vi "generate_DAC_voltages_V1_withPockels.vi"(7 "focus mode?":bool, 8 "derived values":T1, 9 "scan specification":T4={"x amplitude"=0, "x resolution (pixels)"=0, "x offset fly-forward (iterations)"=0, "x offset fly-back (iterations)"=0, "y resolution (nr. of lines)"=0, "y step size"=0, "iterations per pixel"=0, "number of frames"=0, "y offset (pixels)"=0, "number of y-brake lines  (before y-fly-back)"=0, "number y-brake lines (after y-fly-back)"=0, "number of y-fly-back steps"=8, "lines per z step"=0, "number of z/intensity tuples"=0, "number of repetitions (volumes or planes)"=0, "z step size derived"=0, "choose the beginning of z scan"=FALSE, "number of frames (settings)"=0, "FPGA trajectory?"=FALSE, "Pockels cell voltage (bits)"=0}, 10 "counter cluster in":T2, 11 "resonant trigger":bool) -> (0 "acquire?":bool, 1 "fly-back acquisition phase?":bool, 2 "counter cluster out":T2, 3 "DAC voltages":T3 {"ch6" max=4095 step=1; "ch5" max=4095 step=1; "ch4" max=4095 step=1; "ch3" max=4095 step=1; "ch2" max=4095 step=1; "ch1" max=4095 step=1; "ch0" max=4095 step=1})   [LabVIEW 2010]
uses:
  scan_specification_cluster.ctl
  common_typedefs/DAC_voltage_cluster.ctl
  counter_cluster.ctl
  derived_values_cluster.ctl
panel:
  out "coerced(x)":u16
  out "coerced(x) 2":u16
  out "unsigned 16bit integer":u16
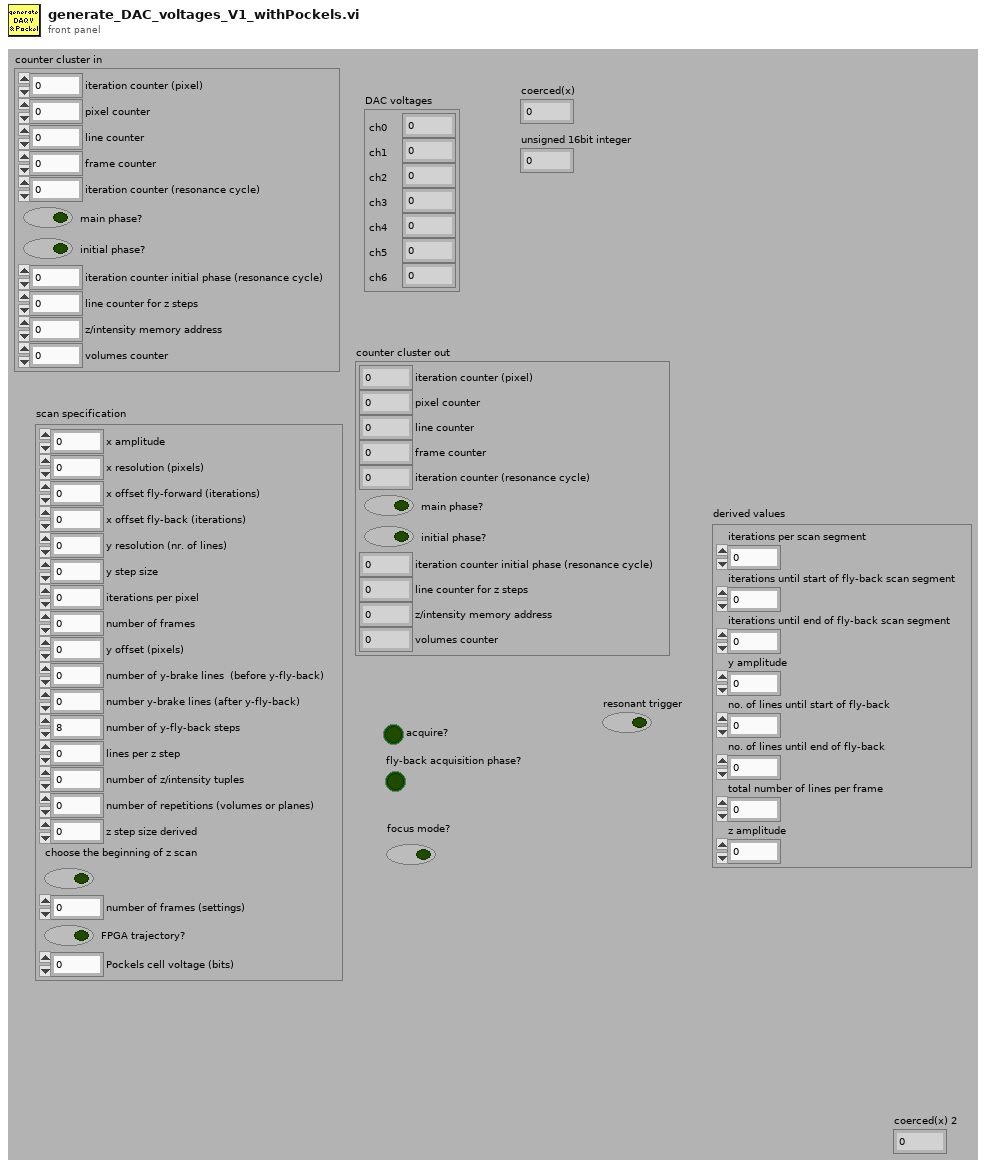
[diagram p1: front panel]
types:
  T1 = typedef "derived_values_cluster.ctl" = cluster{"iterations per scan segment":u16, "iterations until start of fly-back scan segment":u16, "iterations until end of fly-back scan segment":u16, "y amplitude":u16, "no. of lines until start of fly-back":u16, "no. of lines until end of fly-back":u16, "total number of lines per frame ":u16, "z amplitude":u16}
  T2 = typedef "counter_cluster.ctl" = cluster{"iteration counter (pixel)":u16, "pixel counter":u16, "line counter":u16, "frame counter":u16, "iteration counter (resonance cycle)":u16, "main phase?":bool, "initial phase?":bool, "iteration counter initial phase (resonance cycle)":u16, "line counter for z steps":u16, "z/intensity memory address":u32, "volumes counter":u16}
  T3 = typedef "DAC_voltage_cluster.ctl" = cluster{"ch0":u16, "ch1":i16, "ch2":i16, "ch3":i16, "ch4":u16, "ch5":u16, "ch6":u16}
  T4 = typedef "scan_specification_cluster.ctl" = cluster{"x amplitude":u16, "x resolution (pixels)":u16, "x offset fly-forward (iterations)":u16, "x offset fly-back (iterations)":u16, "y resolution (nr. of lines)":u16, "y step size":u16, "iterations per pixel":u16, "number of frames":i32, "y offset (pixels)":u16, "number of y-brake lines  (before y-fly-back)":u16, "number y-brake lines (after y-fly-back)":u16, "number of y-fly-back steps":u16, "lines per z step":u16, "number of z/intensity tuples":u16, "number of repetitions (volumes or planes)":i32, "z step size derived":u16, "choose the beginning of z scan":bool, "number of frames (settings)":i32, "FPGA trajectory?":bool, "Pockels cell voltage (bits)":i16}
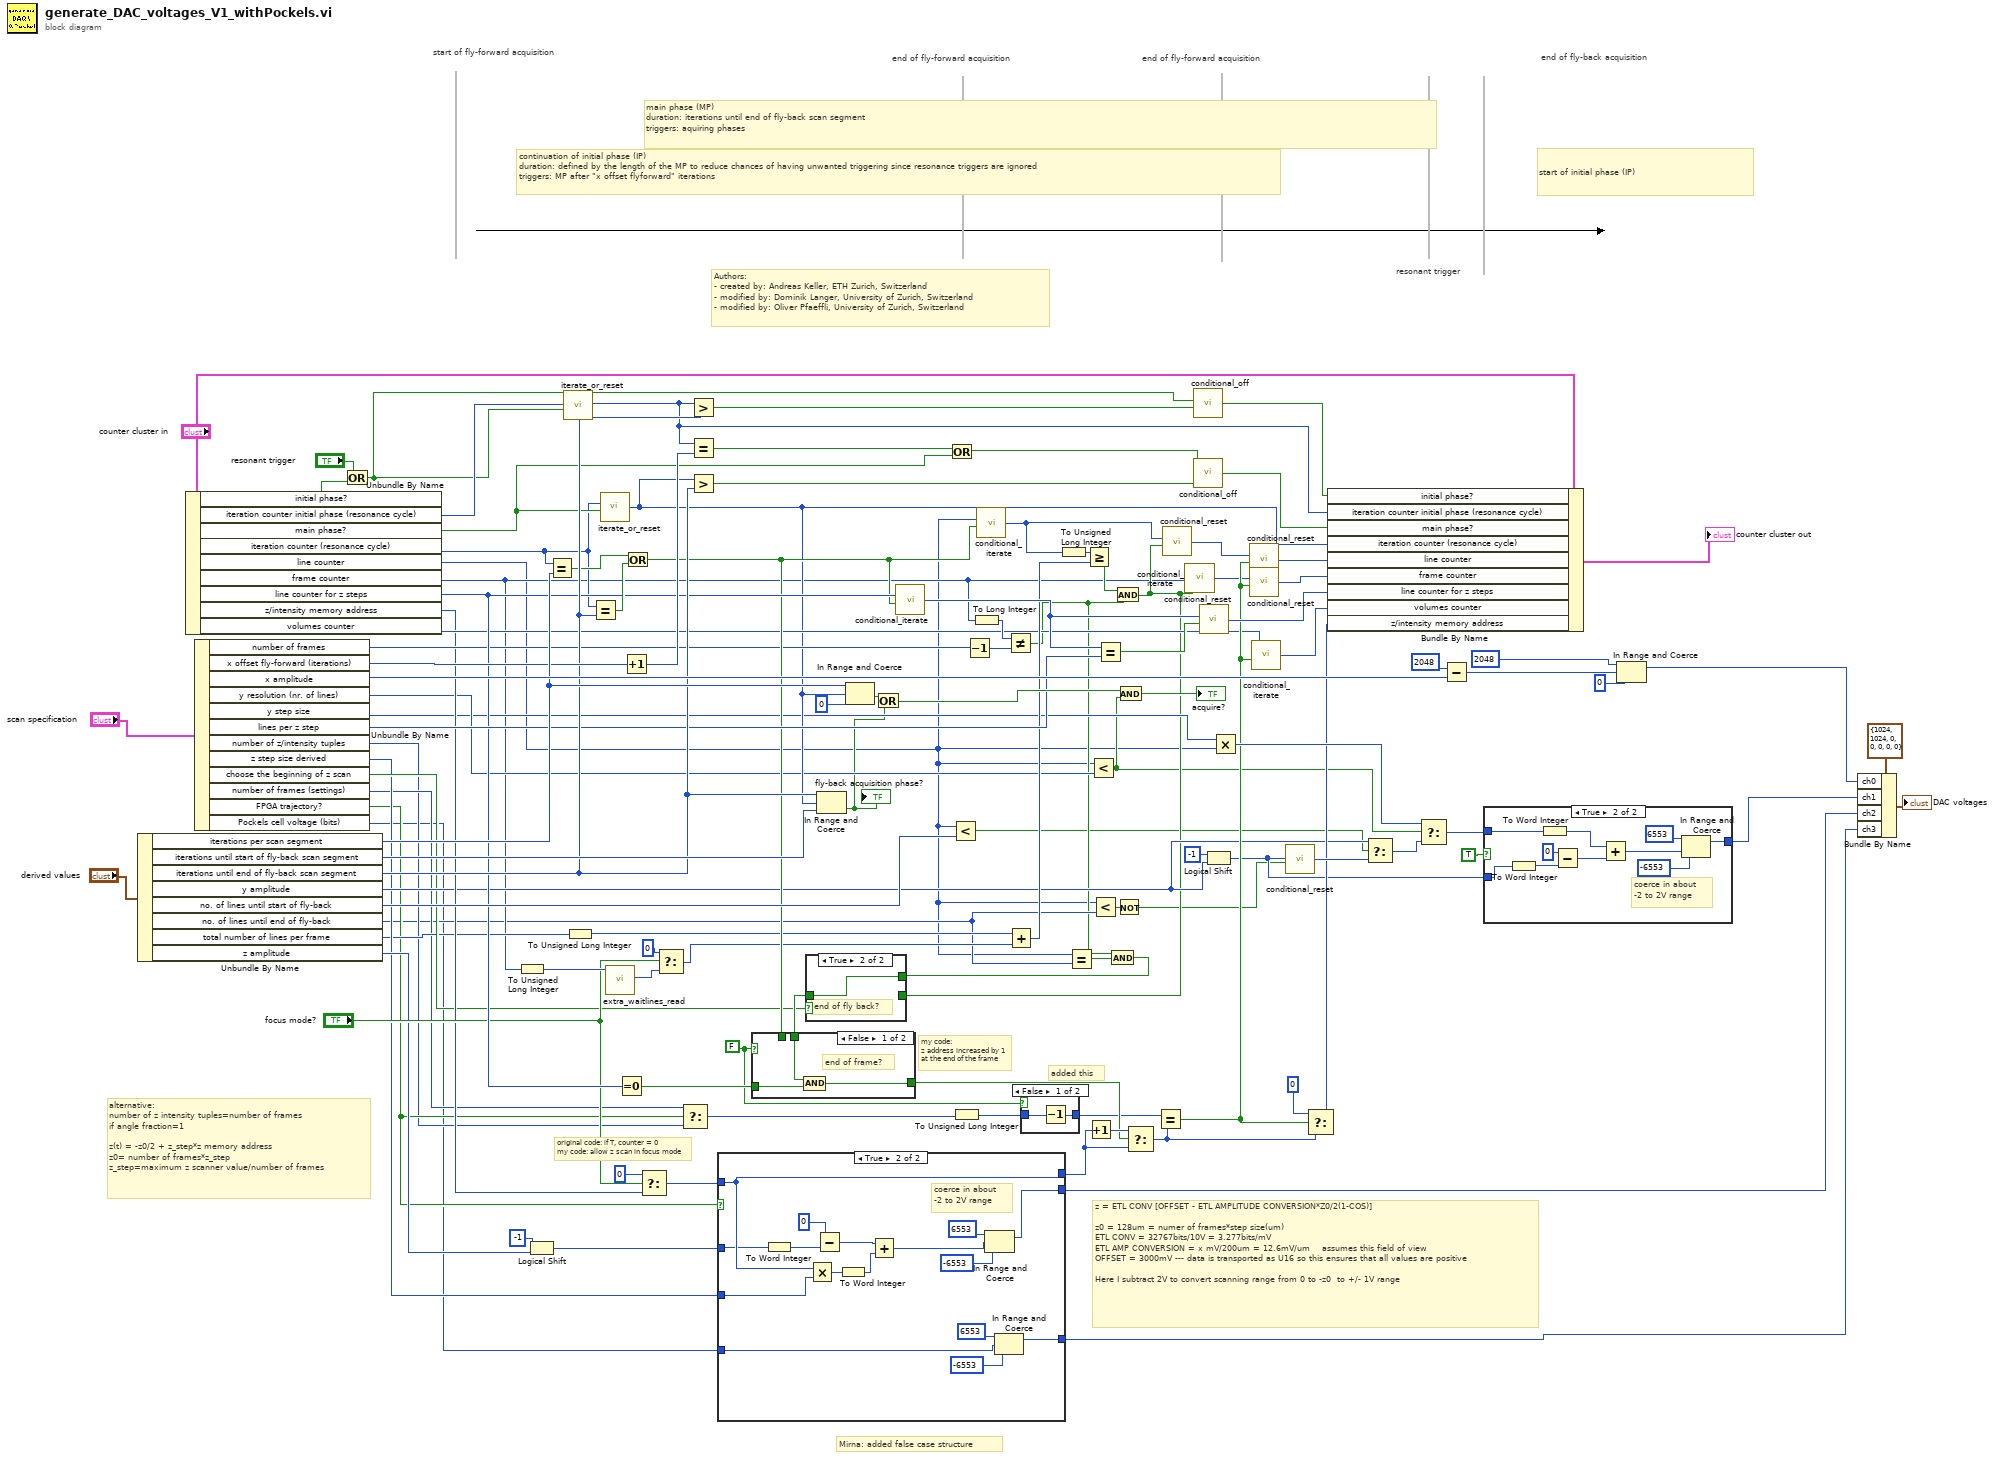
[diagram p0: block diagram]
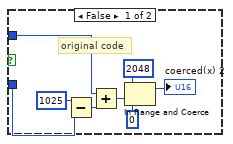
[diagram p3: hidden frame]
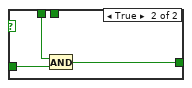
[diagram p5: hidden frame]
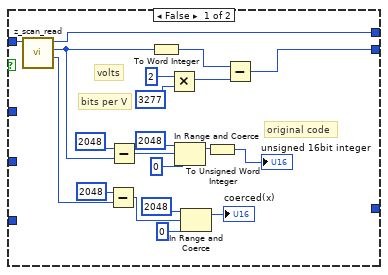
[diagram p6: hidden frame]
diagram:
  w6 = FALSE
  # "added this"
  # "z = ETL CONV [OFFSET - ETL AMPLITUDE CONVERSION*Z0/2(1-COS)]\n\nz0 = 128um = numer of frames*step size(um)\nETL CONV = 32767bits/10V = 3.277bits/mV\nETL AMP CONVERSION = x mV/200um = 12.6mV/um    assumes this field of view\nOFFSET = 3000mV --- data is transported as U16 so this ensures that all values are positive\n\nHere I subtract 2V to convert scanning range from 0 to -z0  to +/- 1V range"
  # "my code:\nz address increased by 1\nat the end of the frame"
  # "alternative:\nnumber of z intensity tuples=number of frames\nif angle fraction=1\n\nz(t) = -z0/2 + z_step*z memory address\nz0= number of frames*z_step\nz_step=maximum z scanner value/number of frames"
  # "original code: if T, counter = 0\nmy code: allow z scan in focus mode"
  # "Mirna: added false case structure"
  # "start of initial phase (IP)"
  # "continuation of initial phase (IP)\nduration: defined by the length of the MP to reduce chances of having unwanted triggering since resonance triggers are ignored\ntriggers: MP after \"x offset flyforward\" iterations"
  # "end of fly-back acquisition"
  # "end of fly-forward acquisition"
  # "end of fly-forward acquisition"
  # "start of fly-forward acquisition"
  # "main phase (MP)\nduration: iterations until end of fly-back scan segment\ntriggers: aquiring phases"
  # "resonant trigger"
  # "Authors: \n- created by: Andreas Keller, ETH Zurich, Switzerland\n- modified by: Dominik Langer, University of Zurich, Switzerland\n- modified by: Oliver Pfaeffli, University of Zurich, Switzerland"
  n1 = Unbundle By Name("derived values") -> ("iterations per scan segment"=w93:u16, "iterations until start of fly-back scan segment"=w96:u16, "iterations until end of fly-back scan segment"=w80:u16, "y amplitude"=w36:u16, "no. of lines until start of fly-back"=w84:u16, "no. of lines until end of fly-back"=w11:u16, "total number of lines per frame"=w29:u16, "z amplitude"=w34:u16)
  n2 = Unbundle By Name("counter cluster in") -> ("initial phase?"=w95:bool, "iteration counter initial phase (resonance cycle)"=w91:u16, "main phase?"=w47:bool, "iteration counter (resonance cycle)"=w39:u16, "line counter"=w5:u16, "frame counter"=w28:u16, "line counter for z steps"=w73:u16, "z/intensity memory address"=w42:u32, "volumes counter"=w52:u16)
  n3 = Unbundle By Name("scan specification") -> ("number of frames"=w59:i32, "x offset fly-forward (iterations)"=w83:u16, "x amplitude"=w100:u16, "y resolution (nr. of lines)"=w40:u16, "y step size"=w35:u16, "lines per z step"=w77:u16, "number of z/intensity tuples"=w13:u16, "z step size derived"=w30:u16, "choose the beginning of z scan"=w31:bool, "number of frames (settings)"=w14:i32, "FPGA trajectory?"=w15:bool, "Pockels cell voltage (bits)"=w1:i16)
  n4 = Or(x="resonant trigger", y=w95) -> (x .or. y?=w89:bool)
  n5 = To Unsigned Long Integer(number=w28) -> (unsigned 32bit integer=w65:u32)
  n6 = Logical Shift(y=i16 -1 ("n"), x=w34) -> (x << y=w49:u16)
  n7 = Equal?(x=w39, y=w93) -> (x = y?=w78:bool)
  n8 = call "iterate_or_reset.vi"("iterate?"=w89, "number in"=w91) -> ("number out"=w25:u16)  [unwired: 4 in]
  n9 = To Unsigned Long Integer(number=w29) -> (unsigned 32bit integer=w26:u32)
  n10 = Equal?(x=w39, y=w80) -> (x = y?=w79:bool)
  n11 = call "iterate_or_reset.vi"("iterate?"=w47, "number in"=w39) -> ("number out"=w46:u16)  [unwired: 4 in]
  n12 = call "extra_waitlines_read.vi"("address extra waitlines IN"=w65) -> ("extra waitline data"=w8:u32)  [unwired: 9 in, 1 out]
  n13 = Equal To 0?(x=w73) -> (x = 0?=w68:bool)
  n14 = Increment(x=w83) -> (x+1=w82:u16)
  n15 = Or(x=w78, y=w79) -> (x .or. y?=w67:bool)
  n16 = Select(t=u32 0, s="focus mode?", f=w42) -> (s? t:f=w43:u32)
  n17 = Select(t=u32 0, s="focus mode?", f=w8) -> (s? t:f=w54:u32)
  n18 = Select(t=w14, s=w15, f=w13) -> (s? t:f=w41:i32)
  n19 = Greater?(x=w25, y=w80) -> (0:w81:bool)
  n20 = Equal?(x=w25, y=w82) -> (x = y?=w90:bool)
  n21 = Greater?(x=w46, y=w80) -> (0:w87:bool)
  n22 = case shown="True" w15 {
    tunnel: [w134 w148] -> w66
    tunnel: [w119 w139] -> w44
    tunnel: w43 -> [w133 w148]
    tunnel: w49 -> [_ w140]
    tunnel: w30 -> [_ w149]
    tunnel: [_ w136] -> w3
    tunnel: w1 -> [_ w135]
    frame False {
      # "bits per V"
      # "volts"
      # "original code"
      n23 = call "z_scan_read.vi"("address in"=w133) -> ("intensity"=w130:u16, "z-value"=w121:i16, "address out"=w134:u32)  [unwired: 8 in]
      n24 = Subtract(x=i16 2048, y=w130) -> (x-y=w127:u16)
      n25 = Subtract(x=i16 2048, y=w121) -> (x-y=w123:i16)
      n26 = To Word Integer(number=w121) -> (16bit integer=w120:i16)
      n27 = Multiply(x=i16 2 ("y"), y=i16 3277) -> (x*y=w117:i16)
      n28 = In Range and Coerce(upper limit=i16 2048, x=w123, lower limit=i16 0) -> (coerced(x)=w124:i16)  [unwired: 1 out]
      n29 = In Range and Coerce(upper limit=u16 2048, x=w127, lower limit=u16 0) -> (coerced(x)=→"coerced(x)":u16)  [unwired: 1 out]
      n30 = To Unsigned Word Integer(number=w124) -> (unsigned 16bit integer=→"unsigned 16bit integer":u16)
      n31 = Subtract(x=w120, y=w117) -> (x-y=w119:i16)
    }
    frame True {
      # "coerce in about\n-2 to 2V range"
      n32 = To Word Integer(number=w140) -> (16bit integer=w145:i16)
      n33 = Multiply(x=w148, y=w149) -> (x*y=w146:u32)
      n34 = Subtract(x=i16 0, y=w145) -> (x-y=w147:i16)
      n35 = To Word Integer(number=w146) -> (16bit integer=w144:i16)
      n36 = Add(x=w147, y=w144) -> (x+y=w141:i16)
      n37 = In Range and Coerce(upper limit=i16 6553, x=w141, lower limit=i16 -6553) -> (coerced(x)=w139:i16)  [unwired: 1 out]
      n38 = In Range and Coerce(upper limit=i16 6553, x=w135, lower limit=i16 -6553) -> (coerced(x)=w136:i16)  [unwired: 1 out]
    }
  }
  n39 = In Range and Coerce(upper limit=w80, x=w46, lower limit=w96) -> (In Range?=w18:bool)  [unwired: 1 out]
  "fly-back acquisition phase?" <- w18
  n40 = In Range and Coerce(upper limit=w93, x=w46, lower limit=u16 0) -> (In Range?=w108:bool)  [unwired: 1 out]
  n41 = Or(x=w108, y=w18) -> (x .or. y?=w99:bool)
  n42 = call "conditional_iterate.vi"("iterate?"=w67, "number in"=w73) -> ("number out"=w74:u16)  [unwired: 4 in]
  n43 = Or(x=w90, y=w47) -> (x .or. y?=w48:bool)
  n44 = Less?(x=w5, y=w84) -> (x < y?=w2:bool)
  n45 = To Unsigned Long Integer(number=w41) -> (unsigned 32bit integer=w71:u32)
  n46 = Decrement(x=w59) -> (x-1=w58:i32)
  n47 = To Long Integer(number=w28) -> (32bit integer=w57:i32)
  n48 = call "conditional_iterate.vi"("iterate?"=w67, "number in"=w5) -> ("number out"=w10:u16)  [unwired: 4 in]
  n49 = Not Equal?(x=w57, y=w58) -> (x != y?=w9:bool)
  n50 = Add(x=w26, y=w54) -> (x+y=w55:u32)
  n51 = case shown="False" w6 {
    tunnel: w71 -> [w152 w153]
    tunnel: [w151 w153] -> w7
    frame False {
      n52 = Decrement(x=w152) -> (x-1=w151:u32)
    }
    frame True {
    }
  }
  n53 = To Unsigned Long Integer(number=w10) -> (unsigned 32bit integer=w12:u32)
  n54 = Equal?(x=w5, y=w11) -> (x = y?=w16:bool)
  n55 = Greater Or Equal?(x=w12, y=w55) -> (x >= y?=w60:bool)
  n56 = Increment(x=w66) -> (x+1=w72:u32)
  n57 = Less?(x=w5, y=w40) -> (x < y?=w21:bool)
  n58 = Less?(x=w5, y=w11) -> (x < y?=w98:bool)
  n59 = Equal?(x=w74, y=w77) -> (x = y?=w75:bool)
  n60 = And(x=w9, y=w16) -> (x .and. y?=w17:bool)
  n61 = And(x=w60, y=w9) -> (x .and. y?=w33:bool)
  n62 = case shown="True" w31 {
    tunnel: w17 -> [_ w155]
    tunnel: w33 -> [w154 _]
    tunnel: [w154 w155] -> w32
    frame False {
      # "end of frame?"
    }
    frame True {
      # "end of fly back?"
    }
  }
  n63 = case shown="False" w6 {
    tunnel: w68 -> [w158 w161]
    tunnel: w67 -> [_ w160]
    tunnel: [w157 w159] -> w27
    tunnel: w32 -> [w156 _]
    frame False {
      # "end of frame?"
      n64 = And(x=w156, y=w158) -> (x .and. y?=w157:bool)
    }
    frame True {
      n65 = And(x=w160, y=w161) -> (x .and. y?=w159:bool)
    }
  }
  n66 = Not(x=w98) -> (.not. x?=w19:bool)
  n67 = And(x=w99, y=w21) -> (x .and. y?=→"acquire?":bool)
  n68 = Select(t=w72, s=w27, f=w66) -> (s? t:f=w70:u32)
  n69 = Equal?(x=w7, y=w70) -> (x = y?=w56:bool)
  n70 = call "conditional_reset.vi"("reset?"=w33, "number in"=w10) -> ("number out"=w62:u16)  [unwired: 4 in]
  n71 = call "conditional_iterate.vi"("iterate?"=w33, "number in"=w28) -> ("number out"=w37:u16)  [unwired: 4 in]
  n72 = call "conditional_off.vi"("switch off?"=w81, "boolean in"=w89) -> ("boolean out"=w88:bool)  [unwired: 4 in]
  n73 = call "conditional_off.vi"("switch off?"=w87, "boolean in"=w48) -> ("boolean out"=w86:bool)  [unwired: 4 in]
  n74 = call "conditional_reset.vi"("reset?"=w75, "number in"=w74) -> ("number out"=w76:u16)  [unwired: 4 in]
  n75 = Logical Shift(y=i16 -1 ("n"), x=w36) -> (x << y=w20:u16)
  n76 = Multiply(x=w35, y=w5) -> (x*y=w113:u16)
  n77 = call "conditional_reset.vi"("reset?"=w56, "number in"=w62) -> ("number out"=w61:u16)  [unwired: 4 in]
  n78 = call "conditional_reset.vi"("reset?"=w56, "number in"=w37) -> ("number out"=w38:u16)  [unwired: 4 in]
  n79 = call "conditional_iterate.vi"("iterate?"=w56, "number in"=w52) -> ("number out"=w63:u16)  [unwired: 4 in]
  n80 = call "conditional_reset.vi"("reset?"=w19, "number in"=w20) -> ("number out"=w85:u16)  [unwired: 4 in]
  n81 = Select(t=u32 0, s=w56, f=w70) -> (s? t:f=w64:u32)
  n82 = Bundle By Name(cluster="counter cluster in", "initial phase?"=w88, "iteration counter initial phase (resonance cycle)"=w25, "main phase?"=w86, "iteration counter (resonance cycle)"=w46, "line counter"=w61, "frame counter"=w38, "line counter for z steps"=w76, "volumes counter"=w63, "z/intensity memory address"=w64) -> (→"counter cluster out":T2)
  n83 = Select(t=w36, s=w2, f=w85) -> (s? t:f=w22:u16)
  n84 = Select(t=w113, s=w21, f=w22) -> (s? t:f=w24:u16)
  n85 = Subtract(x=u16 2048, y=w100) -> (x-y=w104:u16)
  n86 = case shown="True" TRUE {
    tunnel: [_ w172] -> w45
    tunnel: w20 -> [w162 w171]
    tunnel: w24 -> [w163 w170]
    frame False {
      # "original code"
      n87 = Subtract(x=u16 1025, y=w162) -> (x-y=w165:u16)
      n88 = Add(x=w163, y=w165) -> (x+y=w164:u16)
      n89 = In Range and Coerce(upper limit=u16 2048, x=w164, lower limit=u16 0) -> (coerced(x)=→"coerced(x) 2":u16)  [unwired: 1 out]
    }
    frame True {
      # "coerce in about\n-2 to 2V range"
      n90 = To Word Integer(number=w171) -> (16bit integer=w177:i16)
      n91 = To Word Integer(number=w170) -> (16bit integer=w176:i16)
      n92 = Subtract(x=i16 0, y=w177) -> (x-y=w178:i16)
      n93 = Add(x=w176, y=w178) -> (x+y=w173:i16)
      n94 = In Range and Coerce(upper limit=i16 6553, x=w173, lower limit=i16 -6553) -> (coerced(x)=w172:i16)  [unwired: 1 out]
    }
  }
  n95 = In Range and Coerce(upper limit=u16 2048, x=w104, lower limit=u16 0) -> (coerced(x)=w103:u16)  [unwired: 1 out]
  n96 = Bundle By Name(cluster=T3 {"ch0"=1024, "ch1"=1024, "ch2"=0, "ch3"=0, "ch4"=0, "ch5"=0, "ch6"=0} ("DAC voltage"), "ch0"=w103, "ch1"=w45, "ch2"=w44, "ch3"=w3) -> (→"DAC voltages":T3)
